vi "Connection Open.vi"(8 "Error In":errorcluster, 11 "Connection Data In":T1) -> (0 "Error Out":errorcluster, 3 "Connection Data Out":T1)   [LabVIEW 2014, in "MSX-E3701_dll.lvlib"]
doc: "Abre la conexión del Web Server."
uses:
  MSX-E3701_dll.lvlib
  Typedef/Connection Data.ctl
  E:/Repositorio Magnis/INF002/v0/Modules/HAL/Drivers/Sync/ADDI-DATA MSX-E3701/API/MX370x.dll
  MX370x.dll
  E:/Repositorio Magnis/INF002/v0/Modules/HAL/Drivers/Sync/ADDI-DATA MSX-E3701/API/MXCommon.dll
  MXCommon.dll
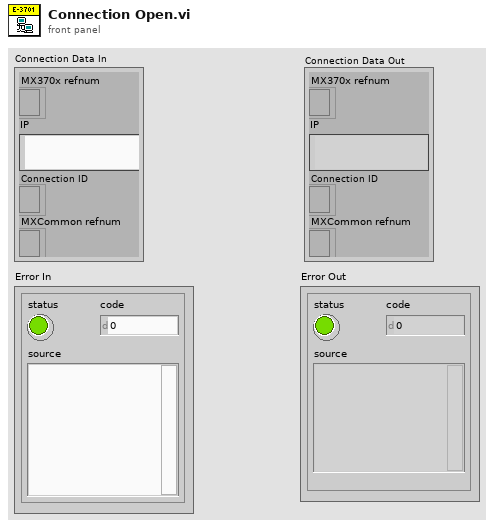
[diagram p1: front panel]
types:
  T1 = typedef "MSX-E3701_dll.lvlib/Connection Data.ctl" = cluster{"MX370x refnum":refnum<k24>, "IP":string, "Connection ID ":refnum<k5>, "MXCommon refnum":refnum<k24>}
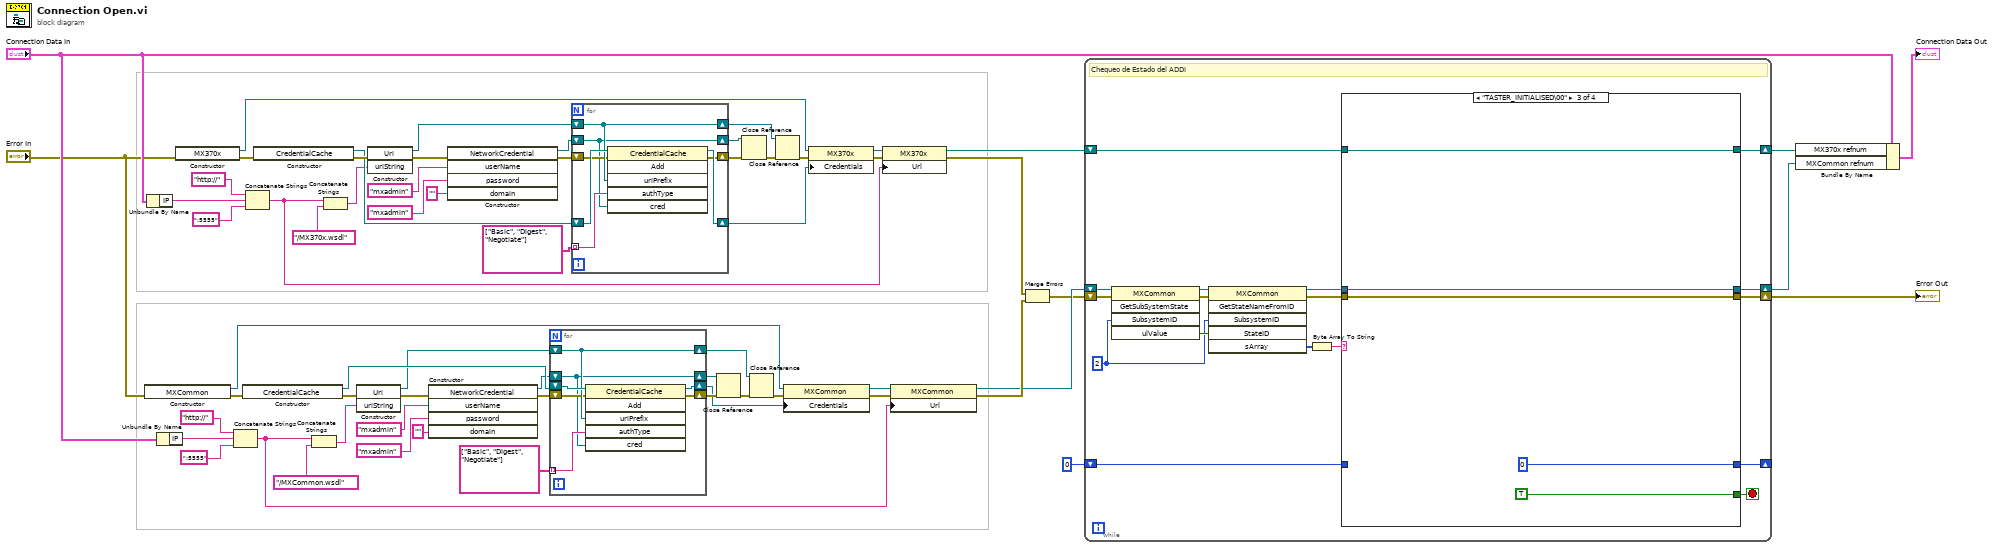
[diagram p0: block diagram]
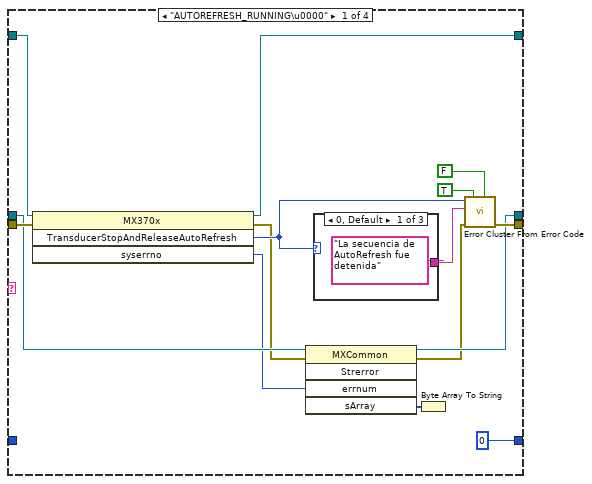
[diagram p2: hidden frame]
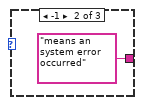
[diagram p3: hidden frame]
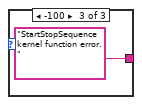
[diagram p4: hidden frame]
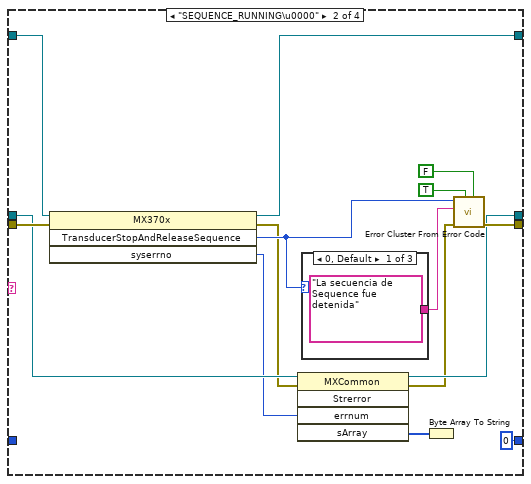
[diagram p5: hidden frame]
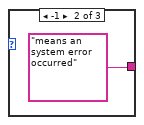
[diagram p6: hidden frame]
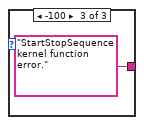
[diagram p7: hidden frame]
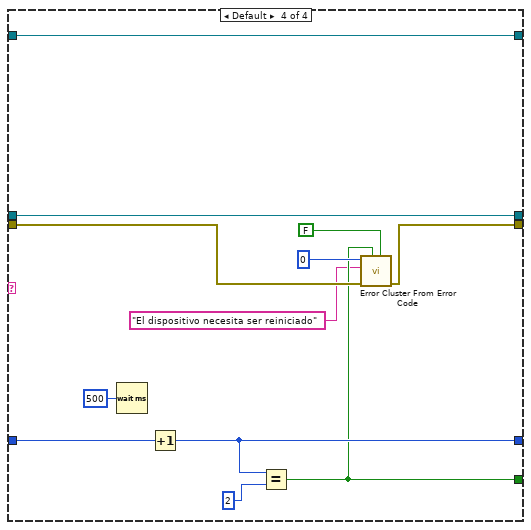
[diagram p8: hidden frame]
diagram:
  n1 = constructor class="MXCommon"(error in="Error In") -> (reference out=w13:refnum<k24>, error out=w12:errorcluster)  [unwired: 2 in, 1 out]
  n2 = Unbundle By Name("Connection Data In") -> ("IP"=w38:string)
  n3 = Unbundle By Name("Connection Data In") -> ("IP"=w19:string)
  n4 = constructor class="MX370x"(error in="Error In") -> (reference out=w64:refnum<k24>, error out=w51:errorcluster)  [unwired: 2 in, 1 out]
  n5 = Concatenate Strings("http://" ("string"), w19, ":5555" ("string")) -> (w16:string)
  n6 = constructor class="CredentialCache"(error in=w12) -> (reference out=w34:refnum<k24>, error out=w37:errorcluster)  [unwired: 2 in, 1 out]
  n7 = Concatenate Strings("http://" ("string"), w38, ":5555" ("string")) -> (w43:string)
  n8 = constructor class="CredentialCache"(error in=w51) -> (reference out=w60:refnum<k24>, error out=w63:errorcluster)  [unwired: 2 in, 1 out]
  n9 = Concatenate Strings(w16, "/MXCommon.wsdl" ("string")) -> (w21:string)
  n10 = Concatenate Strings(w43, "/MX370x.wsdl" ("string")) -> (w41:string)
  n11 = constructor class="Uri"(error in=w37, "uriString"=w21) -> (reference out=w33:refnum<k24>, error out=w36:errorcluster)  [unwired: 2 in, 2 out]
  n12 = constructor class="Uri"(error in=w63, "uriString"=w41) -> (reference out=w59:refnum<k24>, error out=w62:errorcluster)  [unwired: 2 in, 2 out]
  n13 = constructor class="NetworkCredential"(error in=w36, "userName"="mxadmin", "password"="mxadmin" ("userName"), "domain"="" ("userName")) -> (reference out=w32:refnum<k24>, error out=w31:errorcluster)  [unwired: 2 in, 4 out]
  n14 = constructor class="NetworkCredential"(error in=w62, "userName"="mxadmin", "password"="mxadmin" ("userName"), "domain"="" ("userName")) -> (reference out=w58:refnum<k24>, error out=w57:errorcluster)  [unwired: 2 in, 4 out]
  n15 = for {
    tunnel: string[] ["Basic", "Digest", "Negotiate"] -> [w66] mode=indexing
    shift-right: [w67] -> w27
    shift-left: w31 -> [w68]
    shift-right: [w70] -> w29
    shift-left: w33 -> [w70]
    shift-right: [w69] -> w14
    shift-left: w34 -> [w71]
    shift-right: [w65] -> w30
    shift-left: w32 -> [w65]
    n16 = invoke class="CredentialCache" method="Add"(reference=w71, error in=w68, "uriPrefix"=w70, "authType"=w66, "cred"=w65) -> (reference out=w69:refnum<k24>, error out=w67:errorcluster)  [unwired: 1 in, 4 out]
  }
  n17 = for {
    tunnel: string[] ["Basic", "Digest", "Negotiate"] -> [w73] mode=indexing
    shift-right: [w74] -> w53
    shift-left: w57 -> [w75]
    shift-right: [w77] -> w55
    shift-left: w59 -> [w77]
    shift-right: [w76] -> w52
    shift-left: w60 -> [w78]
    shift-right: [w72] -> w56
    shift-left: w58 -> [w72]
    n18 = invoke class="CredentialCache" method="Add"(reference=w78, error in=w75, "uriPrefix"=w77, "authType"=w73, "cred"=w72) -> (reference out=w76:refnum<k24>, error out=w74:errorcluster)  [unwired: 1 in, 4 out]
  }
  n19 = Close Reference(reference=w30, error in (no error)=w27) -> (error out=w28:errorcluster)
  n20 = Close Reference(reference=w56, error in (no error)=w53) -> (error out=w54:errorcluster)
  n21 = Close Reference(reference=w29, error in (no error)=w28) -> (error out=w15:errorcluster)
  n22 = Close Reference(reference=w55, error in (no error)=w54) -> (error out=w50:errorcluster)
  n23 = property class="MXCommon"(reference=w13, error in=w15, "Credentials"=w14) -> (reference out=w18:refnum<k24>, error out=w17:errorcluster)
  n24 = property class="MX370x"(reference=w64, error in=w50, "Credentials"=w52) -> (reference out=w46:refnum<k24>, error out=w45:errorcluster)
  n25 = property class="MX370x"(reference=w46, error in=w45, "Url"=w43) -> (reference out=w5:refnum<k24>, error out=w8:errorcluster)
  n26 = property class="MXCommon"(reference=w18, error in=w17, "Url"=w16) -> (reference out=w7:refnum<k24>, error out=w9:errorcluster)
  n27 = Merge Errors(w8, w9) -> (w6:errorcluster)
  n28 = while {
    shift-right: [w83] -> _
    shift-left: u32 0 ("milliseconds to wait") -> [w84]
    shift-right: [w82] -> w3
    shift-left: w7 -> [w91]
    shift-right: [w81] -> w2
    shift-left: w5 -> [w87]
    shift-right: [w79] -> w1
    shift-left: w6 -> [w89]
    stop <- w85 stop-if-true
    w94 = u64 2 ("SubsystemID 2")
    # "Chequeo de Estado del ADDI"
    n29 = invoke class="MXCommon" method="GetSubSystemState"(reference=w91, error in=w89, "SubsystemID"=w94) -> (reference out=w92:refnum<k24>, error out=w90:errorcluster, "ulValue"=w95:u64)  [unwired: 2 in, 2 out]
    n30 = invoke class="MXCommon" method="GetStateNameFromID"(reference=w92, error in=w90, "SubsystemID"=w94, "StateID"=w95) -> (reference out=w86:refnum<k24>, error out=w80:errorcluster, "sArray"=w93:u8[])  [unwired: 2 in, 3 out]
    n31 = Byte Array To String(unsigned byte array=w93) -> (string=w88:string)
    n32 = case shown="\"TASTER_INITIALISED\\00\"" w88 {
      tunnel: w87 -> [w105 w120 w132 w143]
      tunnel: w86 -> [w100 w119 w134 w144]
      tunnel: [_ _ TRUE w138] -> w85
      tunnel: w84 -> [_ _ _ w146]
      tunnel: [u32 0 u32 0 u32 0 w145] -> w83
      tunnel: [w99 w118 w134 w144] -> w82
      tunnel: [w102 w121 w132 w143] -> w81
      tunnel: w80 -> [w104 w123 w133 w141]
      tunnel: [w103 w122 w133 w140] -> w79
      frame "AUTOREFRESH_RUNNING\u0000" {
        n33 = invoke class="MX370x" method="TransducerStopAndReleaseAutoRefresh"(reference=w105, error in=w104) -> (reference out=w102:refnum<k24>, error out=w97:errorcluster, "TransducerStopAndReleaseAutoRefresh"=w108:i32, "syserrno"=w96:i32)  [unwired: 2 in]
        n34 = invoke class="MXCommon" method="Strerror"(reference=w100, error in=w97, "errnum"=w96) -> (reference out=w99:refnum<k24>, error out=w98:errorcluster, "sArray"=w101:u8[])  [unwired: 2 in, 2 out]
        n35 = case shown="0, Default" w108 {
          tunnel: ["La secuencia de AutoRefresh fue detenida" "means an system error occurred" "StartStopSequence kernel function error."] -> w109
          frame 0, Default {
          }
          frame -1 {
          }
          frame -100 {
          }
        }
        n36 = Byte Array To String(unsigned byte array=w101) -> ()  [unwired: 1 out]
        n37 = call <vilib>:"Error Cluster From Error Code.vi"("is warning? (False)"=FALSE, "show call chain? (False)"=TRUE, "error in (no error)"=w98, "error message (\"\")"=w109, "error code (0)"=w108) -> ("error out"=w103:errorcluster)  [unwired: 4 in]
      }
      frame "SEQUENCE_RUNNING\u0000" {
        n38 = invoke class="MX370x" method="TransducerStopAndReleaseSequence"(reference=w120, error in=w123) -> (reference out=w121:refnum<k24>, error out=w117:errorcluster, "TransducerStopAndReleaseSequence"=w127:i32, "syserrno"=w116:i32)  [unwired: 2 in]
        n39 = invoke class="MXCommon" method="Strerror"(reference=w119, error in=w117, "errnum"=w116) -> (reference out=w118:refnum<k24>, error out=w114:errorcluster, "sArray"=w115:u8[])  [unwired: 2 in, 2 out]
        n40 = case shown="0, Default" w127 {
          tunnel: ["La secuencia de Sequence fue detenida" "means an system error occurred" "StartStopSequence kernel function error."] -> w126
          frame 0, Default {
          }
          frame -1 {
          }
          frame -100 {
          }
        }
        n41 = Byte Array To String(unsigned byte array=w115) -> ()  [unwired: 1 out]
        n42 = call <vilib>:"Error Cluster From Error Code.vi"("is warning? (False)"=FALSE, "show call chain? (False)"=TRUE, "error in (no error)"=w114, "error message (\"\")"=w126, "error code (0)"=w127) -> ("error out"=w122:errorcluster)  [unwired: 4 in]
      }
      frame "TASTER_INITIALISED\u0000" {
      }
      frame Default {
        n43 = Wait (ms)(milliseconds to wait=u32 500) -> ()  [unwired: 1 out]
        n44 = Increment(x=w146) -> (x+1=w145:u32)
        n45 = Equal?(x=w145, y=u32 2 ("milliseconds to wait")) -> (x = y?=w138:bool)
        n46 = call <vilib>:"Error Cluster From Error Code.vi"("is warning? (False)"=FALSE, "show call chain? (False)"=w138, "error in (no error)"=w141, "error message (\"\")"="El dispositivo necesita ser reiniciado", "error code (0)"=0) -> ("error out"=w140:errorcluster)  [unwired: 4 in]
      }
    }
  }
  "Error Out" <- w1
  n47 = Bundle By Name(cluster="Connection Data In", "MX370x refnum"=w2, "MXCommon refnum"=w3) -> (→"Connection Data Out":T1)
